vi "Monitor - Current.vi"(0 "VISA Refnum in":refnum<visa-resource-name>, 5 "Channel":i32, 11 "Error In":errorcluster) -> (4 "VISA Refnum out":refnum<visa-resource-name>, 6 "Current":string, 8 "Current":dbl, 15 "Error Out":errorcluster)   [LabVIEW 2025]
panel:
  out "return count":u32
  out "Command":string
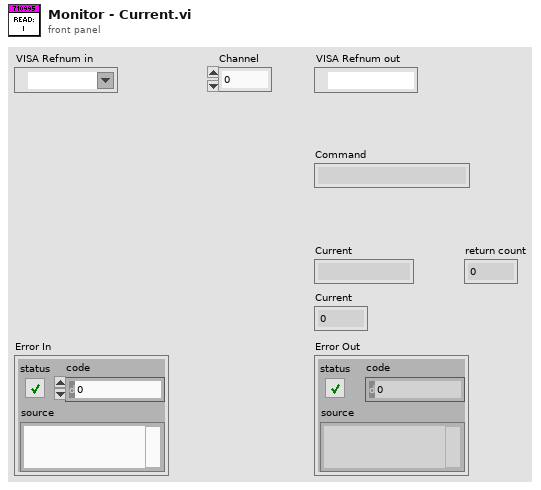
[diagram p1: front panel]
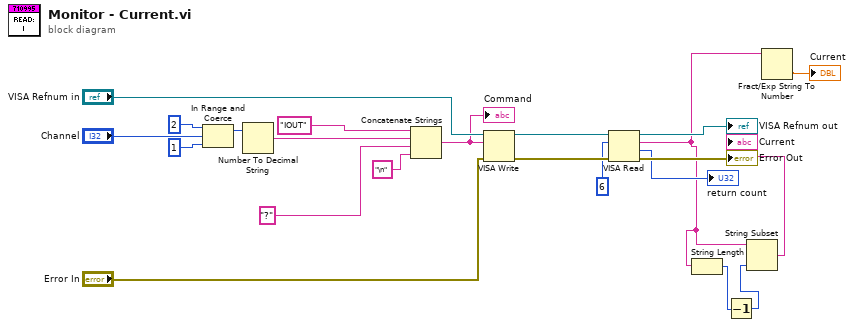
[diagram p0: block diagram]
diagram:
  n1 = In Range and Coerce(upper limit=2, x="Channel", lower limit=1) -> (coerced(x)=w13:i32)  [unwired: 1 out]
  n2 = Number To Decimal String(number=w13) -> (decimal integer string=w15:string)  [unwired: 1 in]
  n3 = Concatenate Strings("IOUT", w15, "?" ("string"), "\n" ("string")) -> (w16:string)
  "Command" <- w16
  n4 = VISA Write(VISA resource name="VISA Refnum in", write buffer=w16, error in (no error)="Error In") -> (VISA resource name out=w18:refnum<visa-resource-name>, error out=w19:errorcluster)  [unwired: 1 out]
  n5 = VISA Read(VISA resource name=w18, byte count=u32 6, error in (no error)=w19) -> (VISA resource name out=→"VISA Refnum out":refnum<visa-resource-name>, read buffer=w3:string, return count=→"return count":u32, error out=→"Error Out":errorcluster)
  n6 = String Length(string=w3) -> (length=w5:i32)
  n7 = Decrement(x=w5) -> (x-1=w4:i32)
  n8 = String Subset(string=w3, length (rest)=w4) -> (substring=→"Current":string)  [unwired: 1 in]
  n9 = Fract/Exp String To Number(string=w3) -> (number=→"Current":dbl)  [unwired: 3 in, 1 out]
